vi "niRFUtil RFHS Compute RMS (complex array).vi"(0 "Complex Array (V)":T1 format="%.2f") -> (4 "RMS (V)":sgl format="%#.2f")   [LabVIEW 2015, in "niRFUtil.lvlib"]
uses:
  niRFUtil.lvlib
  Includes/niRFUtil INC Complex Array.ctl
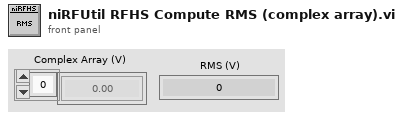
[diagram p1: front panel]
types:
  T1 = typedef "niRFUtil.lvlib/niRFUtil INC Complex Array.ctl" = csg[]
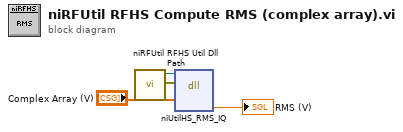
[diagram p0: block diagram]
diagram:
  n1 = call "niRFUtil RFHS Util Dll Path.vi"() -> ("error out"=w3:errorcluster, "Path"=w4:path)  [unwired: 7 in, 3 out]
  n2 = dll-call lib="niRFHS_avx.*" fn="niUtilHS_RMS_IQ"(path in=w4, error in=w3, "iBuf"="Complex Array (V)") -> ("rms"=→"RMS (V)":sgl)  [unwired: 4 in, 2 out]
